vi "SendHistoryPics.vi"(8 "error in (no error)":errorcluster, 11 "TopLevel in":refnum<class "TopLevel.lvclass">) -> (0 "error out":errorcluster, 3 "TopLevel out":refnum<class "TopLevel.lvclass">)   [LabVIEW 2019, in "TopLevel.lvlib" / "TopLevel.lvclass"]
uses:
  TopLevel.lvclass
  TopLevel.lvclass/TopLevel.ctl
  WebSocket/WebSocket Messages/UpdateHistory Msg/UpdateHistory Msg.lvclass/UpdateHistory Msg.ctl
  <vilib>/ActorFramework/Message Enqueuer/Message Enqueuer.lvclass/Message Enqueuer.ctl
  f7a851ff-b167-494b-bc17-cfd5f8a7dee1.vi
  <vilib>/ActorFramework/Message Enqueuer/Enqueue.vi
  WebSocket/WebSocket Messages/UpdateHistory Msg/UpdateHistory Msg.lvclass
  C:/Program Files/National Instruments/LabVIEW 2019/vi.lib/ActorFramework/Message/Message.lvclass
  <vilib>/JDP Science/JSONtext/Variant to JSON Text.vi
  <vilib>/ActorFramework/Message Priority Queue/Priority Enqueue.vi
  <vilib>/JDP Science/JSONtext/LVClass Serializer/JSONtext LVClass Serializer.lvclass
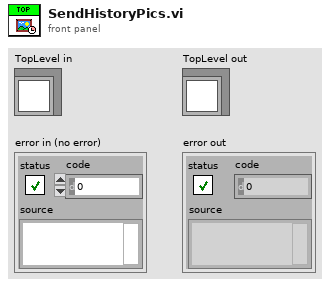
[diagram p1: front panel]
types:
  T1 = typedef "ImageResultModel.ctl" = cluster{"image":string, "pass":bool, "class":string, "time":dbl}
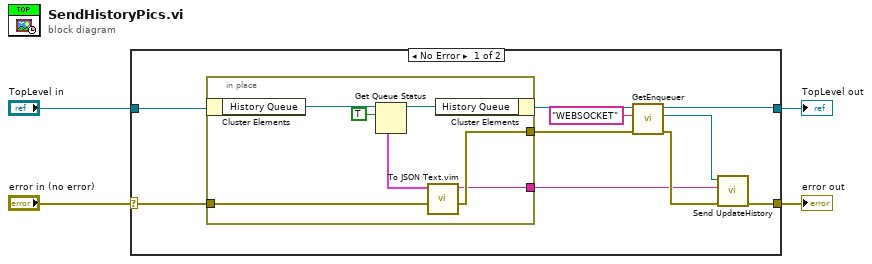
[diagram p0: block diagram]
diagram:
  n1 = case shown="No Error" "error in (no error)" {
    selector: "error in (no error)" -> [w7 w23]
    tunnel: [w5 w23] -> w3
    tunnel: [w6 w22] -> w1
    tunnel: "TopLevel in" -> [w8 w22]
    frame No Error {
      n2 = in-place {
        in-place-border: w7 -> [w17]
        in-place-border: [w16] -> w12
        in-place-border: [w15] -> w9
        n3 = in-place-cluster #1(w8) -> ("History Queue"=w21:refnum<queue>)
        n4 = Get Queue Status(queue=w21, return elements? (F)=TRUE) -> (queue out=w19:refnum<queue>, elements=w18:T1[])  [unwired: 1 in, 6 out]
        n5 = call "To JSON Text.vim"("error in (no error)"=w17, "Anything"=w18) -> ("error out"=w16:errorcluster, "<JSON>"=w15:string)  [unwired: 8 in]
        n6 = in-place-cluster #1("History Queue"=w19) -> (w13:refnum<class "TopLevel.lvclass">)
      }
      n7 = call "GetEnqueuer.vi"("error in (no error)"=w12, "Actor Name"="WEBSOCKET", "TopLevel in"=w13) -> ("error out"=w10:errorcluster, "Enqueuer"=w11:refnum<class "Message Enqueuer.lvclass">, "TopLevel out"=w6:refnum<class "TopLevel.lvclass">)  [unwired: 6 in]
      n8 = call "Send UpdateHistory.vi"("error in (no error)"=w10, "Json Data"=w9, "Message Enqueuer"=w11) -> ("error out"=w5:errorcluster)  [unwired: 7 in, 1 out]
    }
    frame Error {
    }
  }
  "error out" <- w3
  "TopLevel out" <- w1
